vi "check 2d data.vi"(0 "Peak height in":u16[][](array[numeric]), 1 "X input":u16[](array[numeric]), 2 "Y input":u16[](array[numeric]), 5 "time in":u16[][](array[numeric]), 11 "error in (no error)":errorcluster, 12 "X gate input":u16[](array[numeric]), 13 "gate y min":u16[](array[numeric]), 14 "gate y max":u16[](array[numeric])) -> (4 "Peak height out":u16[][](array[numeric]), 6 "time out":u16[][](array[numeric]), 8 "sum of counts out":u32, 15 "error out":errorcluster)   [LabVIEW 2016]
doc: "Vi takes an x and y array of data or time values and determines if they are within a define region for a 2d plot"
uses:
  Drivers/Pixie4DLL.dll
panel:
  out "time before 3":u16[](array[numeric])
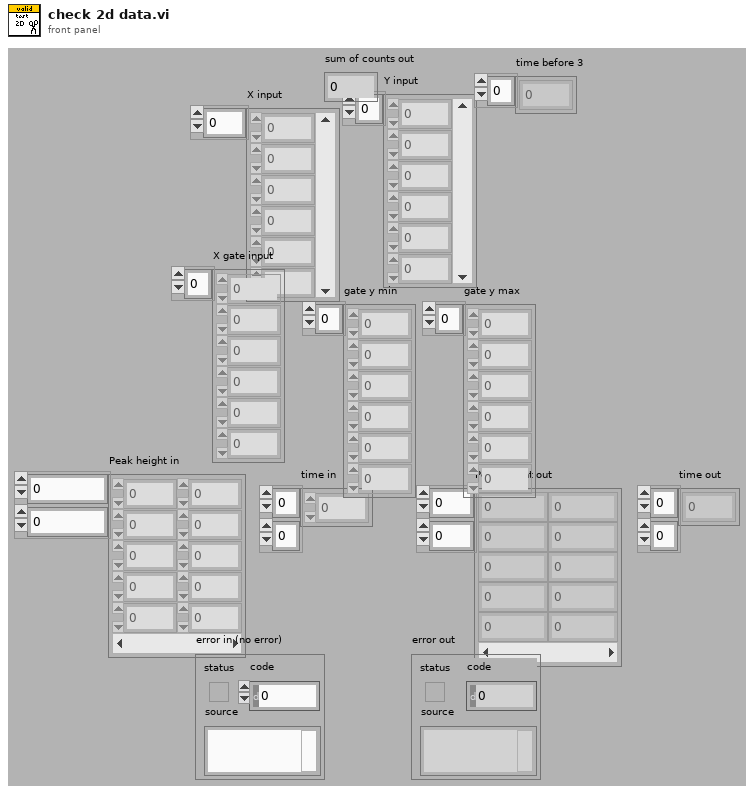
[diagram p1: front panel]
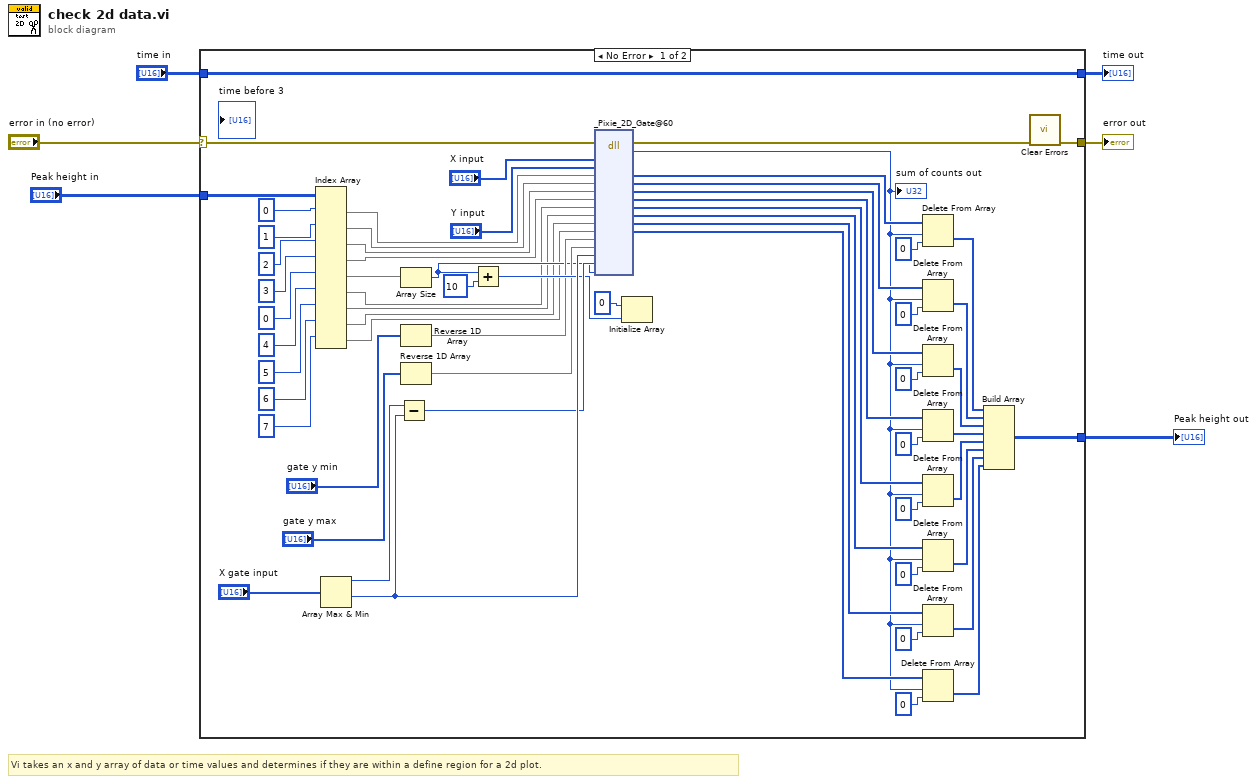
[diagram p0: block diagram]
diagram:
  # "Vi takes an x and y array of data or time values and determines if they are within a define region for a 2d plot."
  n1 = case shown="No Error" "error in (no error)" {
    selector: "error in (no error)" -> [w44 w72]
    tunnel: "time in" -> [w43 w70]
    tunnel: "Peak height in" -> [w55 w71]
    tunnel: [w57 w71] -> w2
    tunnel: [w41 w72] -> w3
    tunnel: [w43 w70] -> w1
    frame No Error {
      n2 = Index Array(array=w55, index (row) #1=0 ("index (row)"), index (row) #2=1 ("index (row)"), index (row) #3=2 ("disabled index (col)"), index (row) #4=3 ("index (row)"), index (row) #5=0 ("index (row)"), index (row) #6=4 ("index (row)"), index (row) #7=5 ("index (row)"), index (row) #8=6 ("index (row)"), index (row) #9=7 ("index (row)")) -> (element #1=w63:u16[], element #2=w66:u16[], element #3=w65:u16[], element #4=w64:u16[], element #5=w45:u16[], element #6=w26:u16[], element #7=w22:u16[], element #8=w21:u16[], element #9=w20:u16[])  [unwired: 9 in]
      n3 = Array Max & Min(array="X gate input") -> (max value=w61:u16, min value=w62:u16)  [unwired: 2 out]
      n4 = Subtract(x=w61, y=w62) -> (x-y=w60:u16)
      n5 = Array Size(array=w45) -> (size(s)=w40:i32)
      n6 = Reverse 1D Array(array="gate y min") -> (reversed array=w48:u16[])
      n7 = Reverse 1D Array(array="gate y max") -> (reversed array=w47:u16[])
      n8 = Add(x=w40, y=u16 10) -> (x+y=w51:i32)
      n9 = dll-call lib="D:/Users/wymanm/Desktop/DAQuiri - 2017a/lois/Drivers/Pixie4DLL.dll" fn="_Pixie_2D_Gate@60"(error in=w44, "X input"="X input", "Y input"="Y input", "datab0"=w63, "datab1"=w66, "datab2"=w65, "datab4"=w64, "timeb1"=w26, "timeb2"=w22, "timeb3"=w21, "timeb4"=w20, "gate y min"=w48, "gate y max"=w47, "offset"=w62, "width"=w60, "number of events"=w40) -> (error out=w42:errorcluster, "return type"=w11:i16, "datab0"=w39:u16[], "datab1"=w36:u16[], "datab2"=w34:u16[], "datab4"=w32:u16[], "timeb1"=w15:u16[], "timeb2"=w14:u16[], "timeb3"=w13:u16[], "timeb4"=w12:u16[])  [unwired: 2 in, 8 out]
      "sum of counts out" <- w11
      n10 = Initialize Array(u32 0 ("index (row)"), w51) -> ()  [unwired: 1 out]
      n11 = Delete From Array(array=w39, length=w11, index=0) -> (deleted portion=w31:u16[])  [unwired: 1 out]
      n12 = Delete From Array(array=w36, length=w11, index=0) -> (deleted portion=w30:u16[])  [unwired: 1 out]
      n13 = Delete From Array(array=w34, length=w11, index=0) -> (deleted portion=w29:u16[])  [unwired: 1 out]
      n14 = Delete From Array(array=w32, length=w11, index=0) -> (deleted portion=w28:u16[])  [unwired: 1 out]
      n15 = Delete From Array(array=w15, length=w11, index=0) -> (deleted portion=w10:u16[])  [unwired: 1 out]
      n16 = Delete From Array(array=w14, length=w11, index=0) -> (deleted portion=w9:u16[])  [unwired: 1 out]
      n17 = Delete From Array(array=w13, length=w11, index=0) -> (deleted portion=w8:u16[])  [unwired: 1 out]
      n18 = Delete From Array(array=w12, length=w11, index=0) -> (deleted portion=w7:u16[])  [unwired: 1 out]
      n19 = Build Array(w31, w30, w29, w28, w10, w9, w8, w7) -> (w57:u16[][])
      n20 = call <vilib>:"Clear Errors.vi"("error in (no error)"=w42) -> ("error out"=w41:errorcluster)  [unwired: 5 in, 1 out]
    }
    frame Error {
    }
  }
  "error out" <- w3
  "Peak height out" <- w2
  "time out" <- w1
